vi "SIM Init Globals.vi"() -> ()   [LabVIEW 2020]
panel:
  in  "RT Solver NaN and Inf Check":bool
  in  "Solver NaN and Inf Check":bool=TRUE
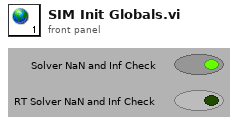
[diagram p1: front panel]
diagram:
